vi "Units_InchesToMeters.vi"(10 "Inches":dbl) -> (2 "Meters":dbl)   [LabVIEW 2019, in "Trajectory_Library.lvlib"]
doc: "Convert a value from inches to meters\n\nInputs: \n - Inches - Distance (Inches)\n\nOutputs:\n - Meters - Distance (Meters)"
uses:
  Trajectory_Library.lvlib
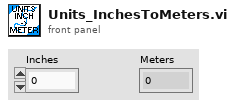
[diagram p1: front panel]
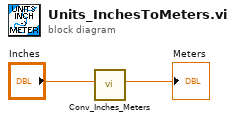
[diagram p0: block diagram]
diagram:
  n1 = call "Conv_Inches_Meters.vi"("INCH"="Inches") -> ("Meters"=→"Meters":dbl)  [unwired: 10 in]
